vi "PKG_IMC_ArcLine_Pos.vi"(0 "handle":u32, 1 "endx":i32, 2 "endy":i32, 3 "cx":i32, 4 "cy":i32, 5 "dir":i32, 6 "pos":i32[](array[numeric])=array[4097 elements], 8 "axisNum":i32, 9 "tgvel":dbl, 10 "endvel":dbl, 11 "wait":i32, 12 "fifo":i32) -> (20 "handle out":u32, 21 "function return":i32, 26 "pos out":i32[](array[numeric]))   [LabVIEW 2011, in "IMC_Pkg4xxx.lvlib"]
doc: "PKG_IMC_ArcLine_Pos(IMC_HANDLE handle, long endx, long endy, long cx, long cy, int dir, long pos[], int axisNum, double tgvel, double endvel, int wait, int fifo);"
uses:
  IMC_Pkg4xxx.lvlib
  IMC_Pkg4xxx.dll
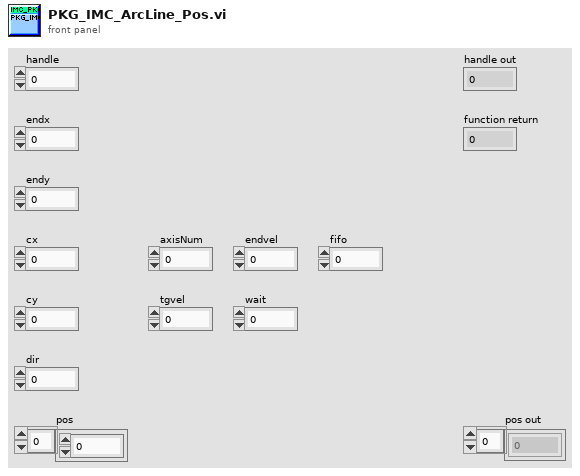
[diagram p1: front panel]
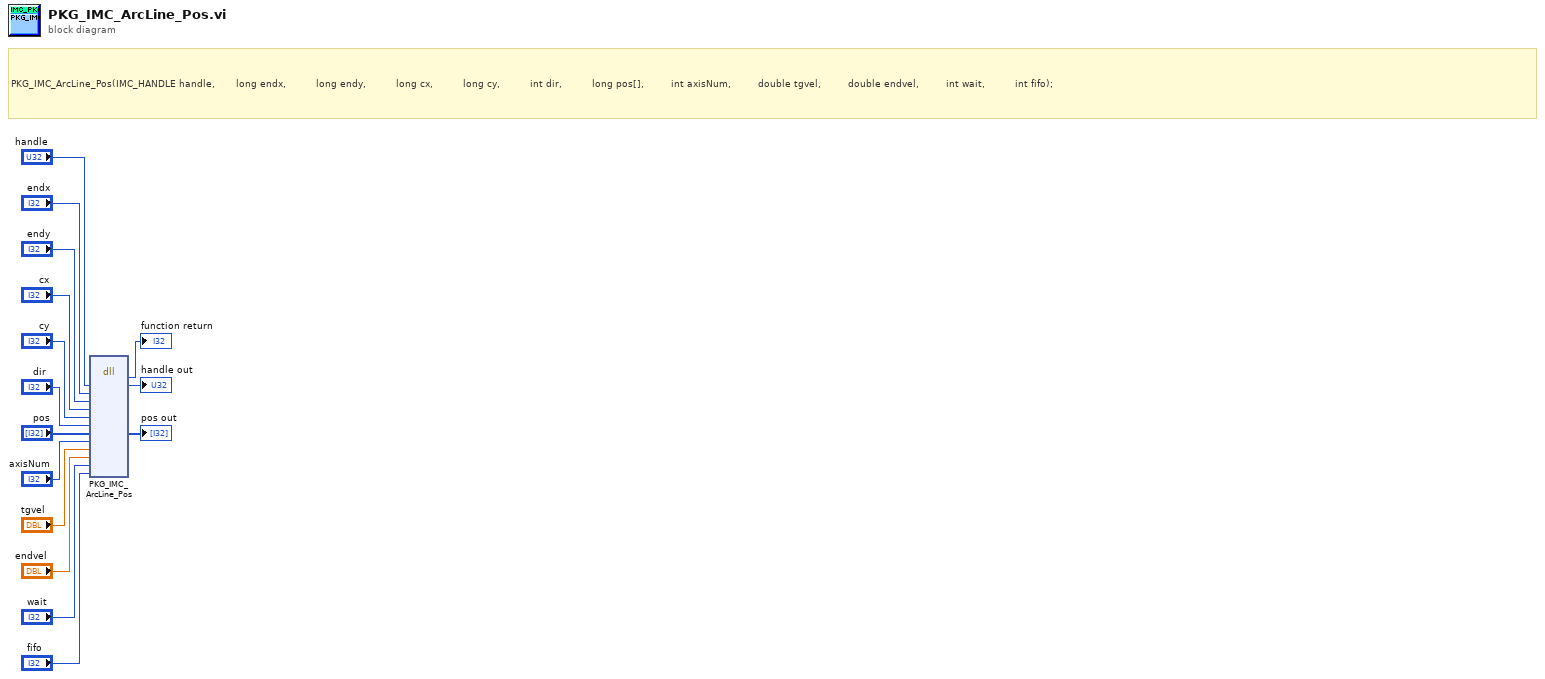
[diagram p0: block diagram]
diagram:
  # "PKG_IMC_ArcLine_Pos(IMC_HANDLE handle, \t\t\t\t\t\tlong endx, \t\t\t\t\t\t\t\t\tlong endy, \t\t\t\t\t\t\t\t\tlong cx, \t\t\t\t\t\t\t\t\tlong cy, \t\t\t\t\t\t\t\t\tint dir, \t\t\t\t\t\t\t\t\tlong pos[], \t\t\t\t\t\t\t\tint axisNum, \t\t\t\t\t\t\t\tdouble tgvel, \t\t\t\t\t\t\t\tdouble endvel, \t\t\t\t\t\t\t\tint wait, \t\t\t\t\t\t\t\t\tint fifo);"
  n1 = dll-call lib="PTH1mabs F光盘刻录\niMC MotionIMCNet_V4.0IMCAppincLabviewIMC_PKG4xxxIMC_PKG4xxx\nIMC_Pkg4xxx.*" fn="PKG_IMC_ArcLine_Pos"("handle"="handle", "endx"="endx", "endy"="endy", "cx"="cx", "cy"="cy", "dir"="dir", "pos"="pos", "axisNum"="axisNum", "tgvel"="tgvel", "endvel"="endvel", "wait"="wait", "fifo"="fifo") -> (→"function return":i32, "handle"=→"handle out":u32, "pos"=→"pos out":i32[])  [unwired: 13 in, 2 out]
